vi "Simon VI.vi"() -> ()   [LabVIEW 2025]
uses:
  color_enums.ctl
  <vilib>/Platform/TimedLoop/XDataNode/timing_clust.ctl
  <vilib>/Platform/TimedLoop/XDataNode/nitl_modes.ctl
  <vilib>/Platform/TimedLoop/XDataNode/wakeup.ctl
  <vilib>/numeric/Random Number (Range) U64.vi
  <vilib>/numeric/sub_Random U32.vi
  <vilib>/platform/TimedLoop/XDataNode/XDataNode.xnode
  <vilib>/Platform/TimedLoop/XDataNode/XDNodeRunTimeDep.lvlib
panel:
  out "Colors":T1
  out "Green":bool
  out "Blue":bool
  out "Purple":bool
  out "Red":bool
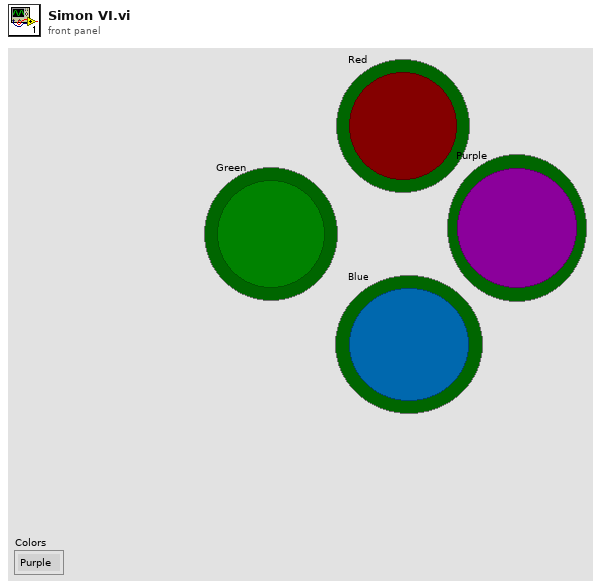
[diagram p1: front panel]
types:
  T1 = typedef "color_enums.ctl" = enum16{"Purple", "Green", "Red", "Blue"}
  T2 = enum16{"Left Button", "Center Button", "Right Button", "Window Close"}
  T3 = typedef "XDNodeRunTimeDep.lvlib/timing_clust.ctl" = cluster{"Expected End [f-1]":u64, "Actual End [f-1]":u64, "Finished Late? [f-1]":bool, "Expected End [i-1]":u64, "Actual End [i-1]":u64, "Finished Late? [i-1]":bool, "Expected Start [i]":u64, "Actual Start [i]":u64, "Expected Start [f]":u64, "Actual Start [f]":u64, "Source Name":string, "Structure Name":string, "Period":i64, "Deadline":i64, "Offset":i64, "Start":i64, "Priority":i32, "Timeout":i32, "Mode":T4, "Wakeup Reason":T5, "Error":errorcluster, "Source Type":string, "Secondary Source Type":string, "Global End Time":u64, "Global Start Time":u64, "Frame Duration":u64, "Iteration Duration":u64, "Assigned CPU":i32, "I/O Scan Engine Mode":u32}
  T4 = typedef "XDNodeRunTimeDep.lvlib/nitl_modes.ctl" = enum32{"No Change", "Process missed periods, maintain original phase", "Discard missed periods, maintain original phase", "Process missed periods, ignore original phase", "Discard missed periods, ignore original phase"}
  T5 = typedef "XDNodeRunTimeDep.lvlib/wakeup.ctl" = enum32{"Normal", "Aborted", "Asynchronous wakeup", "Timing source error", "Timed loop error", "Timeout"}
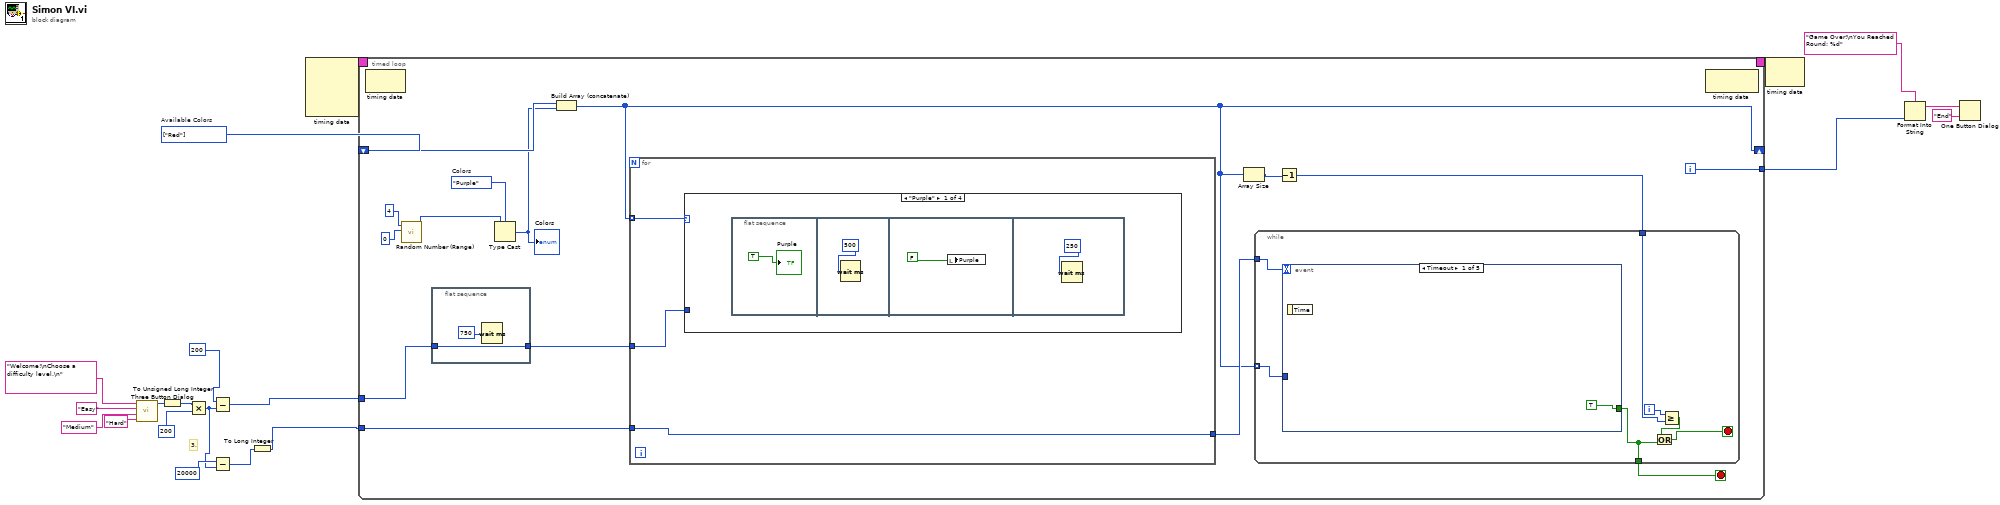
[diagram p0: block diagram]
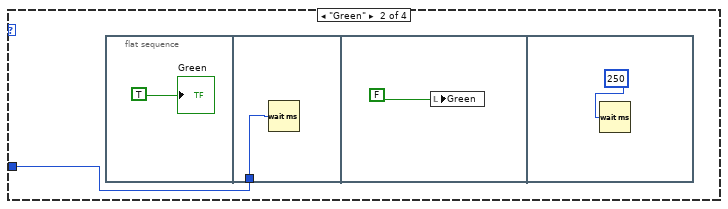
[diagram p2: hidden frame]
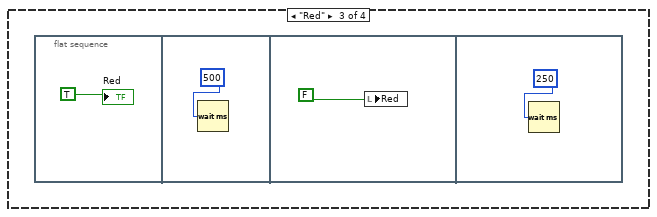
[diagram p3: hidden frame]
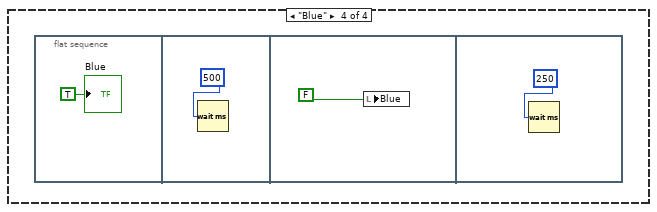
[diagram p4: hidden frame]
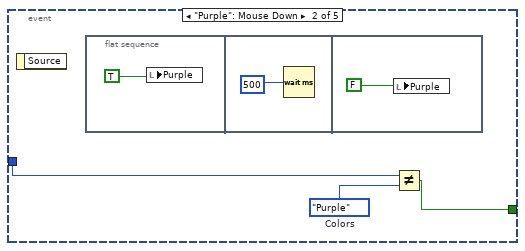
[diagram p5: hidden frame]
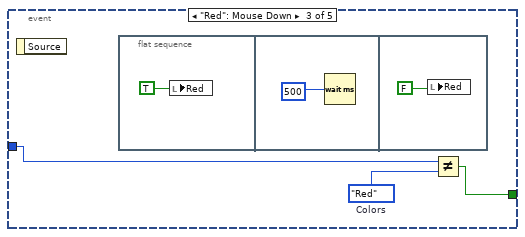
[diagram p6: hidden frame]
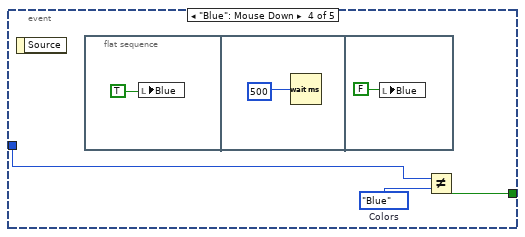
[diagram p7: hidden frame]
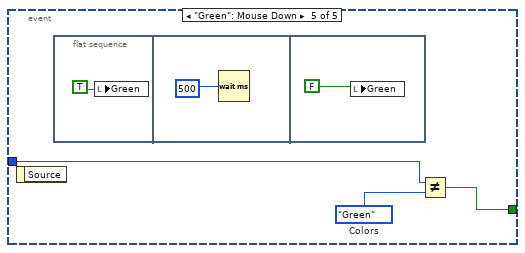
[diagram p8: hidden frame]
diagram:
  w18 = T1[] [enum."Red"] items=["Purple", "Green", "Red", "Blue"]  # Available Colors
  # "3."
  n1 = call <vilib>:"Three Button Dialog.vi"("Right Button Text (\"Cancel\")"="Hard" ("Right Button Text (\"Cancel\")"), "Center Button Text (\"No\")"="Medium" ("Center Button Text (\"No\")"), "Left Button Text (\"Yes\")"="Easy" ("Left Button Text (\"Yes\")"), "message"="Welcome!\nChoose a difficulty level.\n") -> ("Which Button?"=w15:T2)  [unwired: 7 in]
  n2 = To Unsigned Long Integer(number=w15) -> (unsigned 32bit integer=w12:u32)
  n3 = Multiply(x=w12, y=u32 200) -> (x*y=w5:u32)
  n4 = Subtract(x=u32 200, y=w5) -> (x-y=w7:u32)
  n5 = Subtract(x=u32 20000, y=w5) -> (x-y=w9:u32)
  n6 = To Long Integer(number=w9) -> (32bit integer=w8:i32)
  n7 = node-c288() -> (w20:T3)  [unwired: 4 in]
  n8 = timed-loop {
    timing: w20 -> [_]
    timing-out: [_] -> w19
    shift-right: [w28] -> _
    shift-left: w18 -> [w35]
    tunnel: w8 -> [w33]
    tunnel: w7 -> [w32]
    tunnel: [w24] -> w1
    i -> [w24]
    stop <- w25 stop-if-true
    w27 = color_enums."Purple"  # Colors
    n9 = node-c288() -> ()  [unwired: 1 in, 1 out]
    n10 = call-poly <vilib>:"Random Number (Range).vi"("lower bound (0)"=u64 0, "upper bound (100)"=u64 4) -> ("number"=w23:u64)  [unwired: 9 in]
    n11 = flat-sequence {
      tunnel: [w89] -> w31
      tunnel: w32 -> [w89]
      frame #0 {
        n12 = Wait (ms)(milliseconds to wait=u32 750 ("millisecond multiple")) -> ()  [unwired: 1 out]
      }
    }
    n13 = Type Cast(type=w27, x=w23) -> (*(type *) &x=w26:T1)
    "Colors" <- w26
    n14 = Build Array (concatenate)(w35, w26) -> (w28:T1[])
    n15 = for {
      tunnel: w28 -> [w38] mode=indexing
      tunnel: [w37] -> w34
      tunnel: w33 -> [w37]
      tunnel: w31 -> [w36]
      n16 = case shown="\"Purple\"" w38 {
        tunnel: w36 -> [_ w43 _ _]
        frame "Purple" {
          n17 = flat-sequence {
            frame #0 {
              "Purple" <- TRUE
            }
            frame #1 {
              n18 = Wait (ms)(milliseconds to wait=u32 500) -> ()  [unwired: 1 out]
            }
            frame #2 {
              n19 = local write "Purple"(FALSE) -> ()
            }
            frame #3 {
              n20 = Wait (ms)(milliseconds to wait=u32 250) -> ()  [unwired: 1 out]
            }
          }
        }
        frame "Green" {
          n21 = flat-sequence {
            tunnel: w43 -> [w45]
            frame #0 {
              "Green" <- TRUE
            }
            frame #1 {
              n22 = Wait (ms)(milliseconds to wait=w45) -> ()  [unwired: 1 out]
            }
            frame #2 {
              n23 = local write "Green"(FALSE) -> ()
            }
            frame #3 {
              n24 = Wait (ms)(milliseconds to wait=u32 250) -> ()  [unwired: 1 out]
            }
          }
        }
        frame "Red" {
          n25 = flat-sequence {
            frame #0 {
              "Red" <- TRUE
            }
            frame #1 {
              n26 = Wait (ms)(milliseconds to wait=u32 500) -> ()  [unwired: 1 out]
            }
            frame #2 {
              n27 = local write "Red"(FALSE) -> ()
            }
            frame #3 {
              n28 = Wait (ms)(milliseconds to wait=u32 250) -> ()  [unwired: 1 out]
            }
          }
        }
        frame "Blue" {
          n29 = flat-sequence {
            frame #0 {
              "Blue" <- TRUE
            }
            frame #1 {
              n30 = Wait (ms)(milliseconds to wait=u32 500) -> ()  [unwired: 1 out]
            }
            frame #2 {
              n31 = local write "Blue"(FALSE) -> ()
            }
            frame #3 {
              n32 = Wait (ms)(milliseconds to wait=u32 250) -> ()  [unwired: 1 out]
            }
          }
        }
      }
    }
    n33 = Array Size(array=w28) -> (size(s)=w30:i32)
    n34 = Decrement(x=w30) -> (x-1=w29:i32)
    n35 = while {
      tunnel: w34 -> [w62]
      tunnel: w29 -> [w61]
      tunnel: w28 -> [w59] mode=indexing
      tunnel: [w56] -> w25
      i -> [w60]
      stop <- w57 stop-if-true
      n36 = event shown="[0] Timeout" {
        selector: _ -> [_ _ _ _ _]
        dyn-events: _ -> [_ _ _ _ _]
        timeout: w62 -> [_ _ _ _ _]
        tunnel: [TRUE w66 w70 w77 w83] -> w56
        tunnel: w59 -> [_ w64 w71 w76 w82]
        event Timeout {
          n37 = event-data() -> ()  [unwired: 1 in, 1 out]
        }
        event "Purple": Mouse Down {
          w65 = color_enums."Purple"  # Colors
          n38 = event-data() -> ()  [unwired: 1 in, 1 out]
          n39 = flat-sequence {
            frame #0 {
              n40 = local write "Purple"(TRUE) -> ()
            }
            frame #1 {
              n41 = Wait (ms)(milliseconds to wait=u32 500) -> ()  [unwired: 1 out]
            }
            frame #2 {
              n42 = local write "Purple"(FALSE) -> ()
            }
          }
          n43 = Not Equal?(x=w64, y=w65) -> (x != y?=w66:bool)
        }
        event "Red": Mouse Down {
          w72 = color_enums."Red"  # Colors
          n44 = event-data() -> ()  [unwired: 1 in, 1 out]
          n45 = flat-sequence {
            frame #0 {
              n46 = local write "Red"(TRUE) -> ()
            }
            frame #1 {
              n47 = Wait (ms)(milliseconds to wait=u32 500) -> ()  [unwired: 1 out]
            }
            frame #2 {
              n48 = local write "Red"(FALSE) -> ()
            }
          }
          n49 = Not Equal?(x=w71, y=w72) -> (x != y?=w70:bool)
        }
        event "Blue": Mouse Down {
          w78 = color_enums."Blue"  # Colors
          n50 = event-data() -> ()  [unwired: 1 in, 1 out]
          n51 = flat-sequence {
            frame #0 {
              n52 = local write "Blue"(TRUE) -> ()
            }
            frame #1 {
              n53 = Wait (ms)(milliseconds to wait=u32 500) -> ()  [unwired: 1 out]
            }
            frame #2 {
              n54 = local write "Blue"(FALSE) -> ()
            }
          }
          n55 = Not Equal?(x=w76, y=w78) -> (x != y?=w77:bool)
        }
        event "Green": Mouse Down {
          w84 = color_enums."Green"  # Colors
          n56 = event-data() -> ()  [unwired: 1 in, 1 out]
          n57 = flat-sequence {
            frame #0 {
              n58 = local write "Green"(TRUE) -> ()
            }
            frame #1 {
              n59 = Wait (ms)(milliseconds to wait=u32 500) -> ()  [unwired: 1 out]
            }
            frame #2 {
              n60 = local write "Green"(FALSE) -> ()
            }
          }
          n61 = Not Equal?(x=w82, y=w84) -> (x != y?=w83:bool)
        }
      }
      n62 = Greater Or Equal?(x=w60, y=w61) -> (x >= y?=w58:bool)
      n63 = Or(x=w58, y=w56) -> (x .or. y?=w57:bool)
    }
    n64 = node-c288() -> ()  [unwired: 1 in, 1 out]
  }
  n65 = node-c288(w19) -> ()  [unwired: 1 out]
  n66 = Format Into String(format string="Game Over!\nYou Reached Round: %d" ("initial string"), w1) -> (resulting string=w2:string)  [unwired: 2 in, 1 out]
  n67 = One Button Dialog(message=w2, button name ("OK")="End") -> ()  [unwired: 1 out]
